vi "Set VISA资源名称.vi"(10 "VISA资源名称":refnum<visa-resource-name>, 11 "EPEVER-MPPT in":refnum<class "EPEVER-MPPT.lvclass">) -> (3 "EPEVER-MPPT out":refnum<class "EPEVER-MPPT.lvclass">)   [LabVIEW 2016, in "EPEVER-MPPT.lvlib" / "EPEVER-MPPT.lvclass"]
uses:
  EPEVER-MPPT.lvclass
  EPEVER-MPPT.lvclass/EPEVER-MPPT.ctl
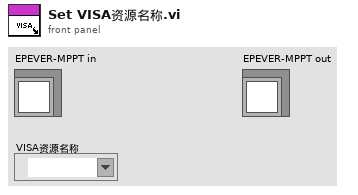
[diagram p1: front panel]
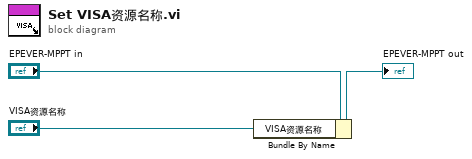
[diagram p0: block diagram]
diagram:
  n1 = Bundle By Name(cluster="EPEVER-MPPT in", "VISA资源名称"="VISA资源名称") -> (→"EPEVER-MPPT out":refnum<class "EPEVER-MPPT.lvclass">)
